vi "Clear Process.vi"(8 "error in (no error)":errorcluster, 11 "Process Executor in":refnum<class "Process Executor.lvclass">) -> (0 "error out":errorcluster, 3 "Process Executor out":refnum<class "Process Executor.lvclass">)   [LabVIEW 2025, in "Process Executor.lvclass"]
doc: "Closes references to a process and its start information object, then clears related data in the process executor object."
uses:
  Process Executor.lvclass
  Process Executor.lvclass/Process Executor.ctl
  Type Definitions/Execution Plan--cluster.ctl
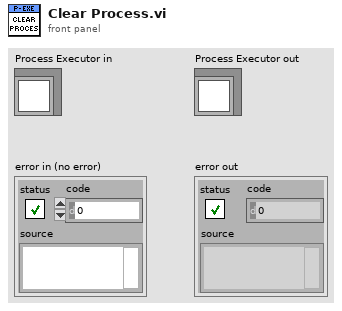
[diagram p1: front panel]
types:
  T1 = typedef "Execution Plan--cluster.ctl" = cluster{"Exe Path":path, "Args":string[], "Timeout":i32}
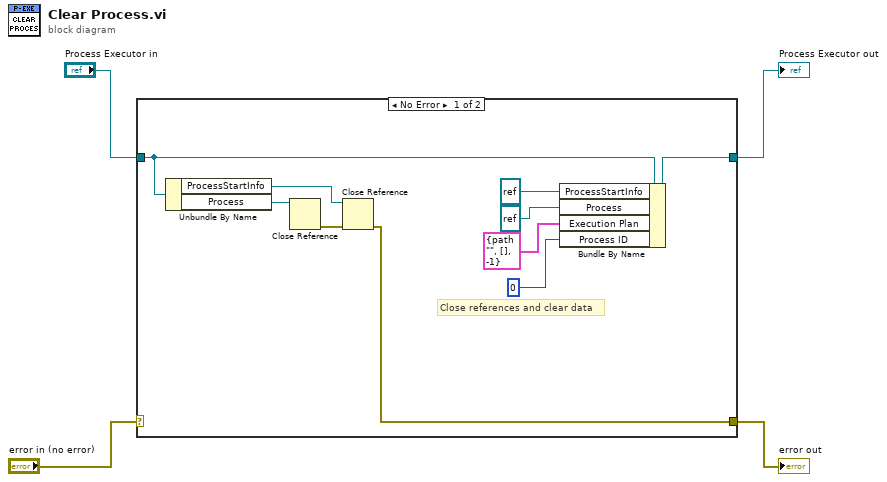
[diagram p0: block diagram]
diagram:
  n1 = case shown="No Error" "error in (no error)" {
    selector: "error in (no error)" -> [_ w16]
    tunnel: [w11 w16] -> w3
    tunnel: [w10 w15] -> w1
    tunnel: "Process Executor in" -> [w9 w15]
    frame No Error {
      # "Close references and clear data"
      n2 = Unbundle By Name(w9) -> ("ProcessStartInfo"=w12:refnum<k39>, "Process"=w14:refnum<k39>)
      n3 = Close Reference(reference=w14) -> (error out=w13:errorcluster)  [unwired: 1 in]
      n4 = Close Reference(reference=w12, error in (no error)=w13) -> (error out=w11:errorcluster)
      n5 = Bundle By Name(cluster=w9, "ProcessStartInfo"=refnum<k39> refnum, "Process"=refnum<k39> refnum, "Execution Plan"=T1 {"Exe Path"=path "", "Args"=[], "Timeout"=-1}, "Process ID"=0) -> (w10:refnum<class "Process Executor.lvclass">)
    }
    frame Error {
    }
  }
  "error out" <- w3
  "Process Executor out" <- w1
